vi "Save Window Position and Size.vi"(8 "error in":errorcluster, 10 "NewBnds":T1) -> (0 "error out":errorcluster)   [LabVIEW 2019, in "Panther Dashboard.lvlib"]
uses:
  <vilib>/Utility/miscctls.llb/LVRectTypeDef.ctl
  <vilib>/Utility/config.llb/Write Key (String).vi
  Panther Dashboard.lvlib
  <vilib>/Utility/config.llb/NI_LVConfig.lvlib
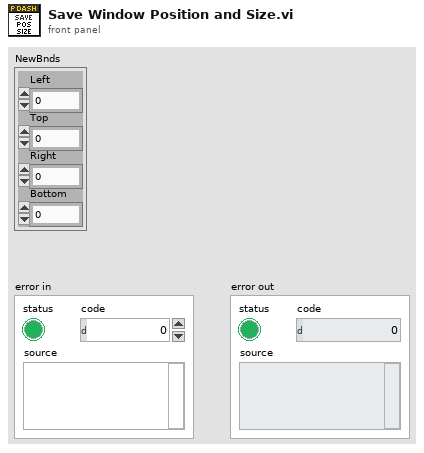
[diagram p1: front panel]
types:
  T1 = typedef "LVRectTypeDef.ctl" = cluster{"Left":i16, "Top":i16, "Right":i16, "Bottom":i16}
  T2 = typedef "NI_LVConfig.lvlib/Config Data RefNum.ctl" = refnum<k1>
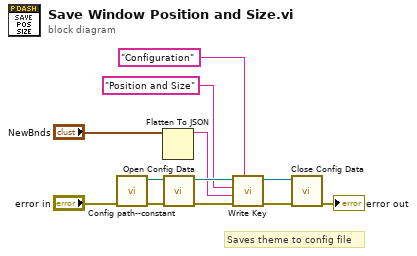
[diagram p0: block diagram]
diagram:
  # "Saves theme to config file"
  n1 = call "Config path--constant.vi"("error in (no error)"="error in") -> ("error out"=w9:errorcluster, "Config Path"=w3:path)  [unwired: 9 in]
  n2 = Flatten To JSON(anything="NewBnds") -> (JSON string=w1:string)  [unwired: 2 in, 1 out]
  n3 = call <vilib>:"Open Config Data.vi"("error in (no error)"=w9, "configuration file path"=w3) -> ("error out"=w10:errorcluster, "refnum"=w6:T2)  [unwired: 7 in, 1 out]
  n4 = call-poly <vilib>:"Write Key.vi"("section"="Configuration", "error in (no error)"=w10, "value"=w1, "key"="Position and Size", "refnum"=w6) -> ("error out"=w11:errorcluster, "refnum out"=w7:T2)  [unwired: 4 in, 1 out]
  n5 = call <vilib>:"Close Config Data.vi"("error in (no error)"=w11, "refnum"=w7) -> ("error out"=→"error out":errorcluster)  [unwired: 8 in, 1 out]
